vi "Motion@WaitPathIndex__Parameter.vi"(1 "ParamterIn":string) -> (0 "ParamterOut":string)   [LabVIEW 2020]
panel:
  in  "Message=":string(combo)
  in  "TimeOut=":string(combo)
  in  "Parameter":string(combo)
  in  "MotorName":string(combo)
  in  "Confirm":bool
  # "Motion@WaitPathIndex $Motor,$Index(,TimeOut=XXX,Message=XXX)"
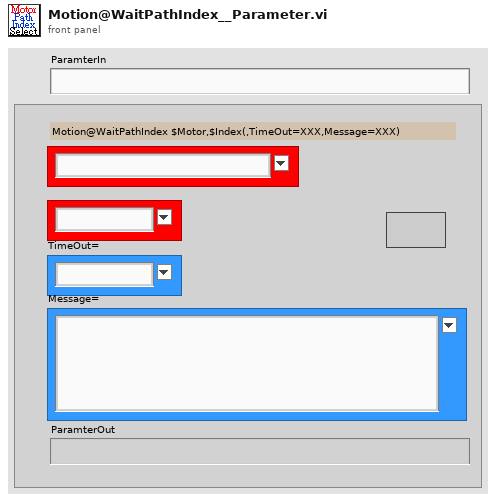
[diagram p1: front panel]
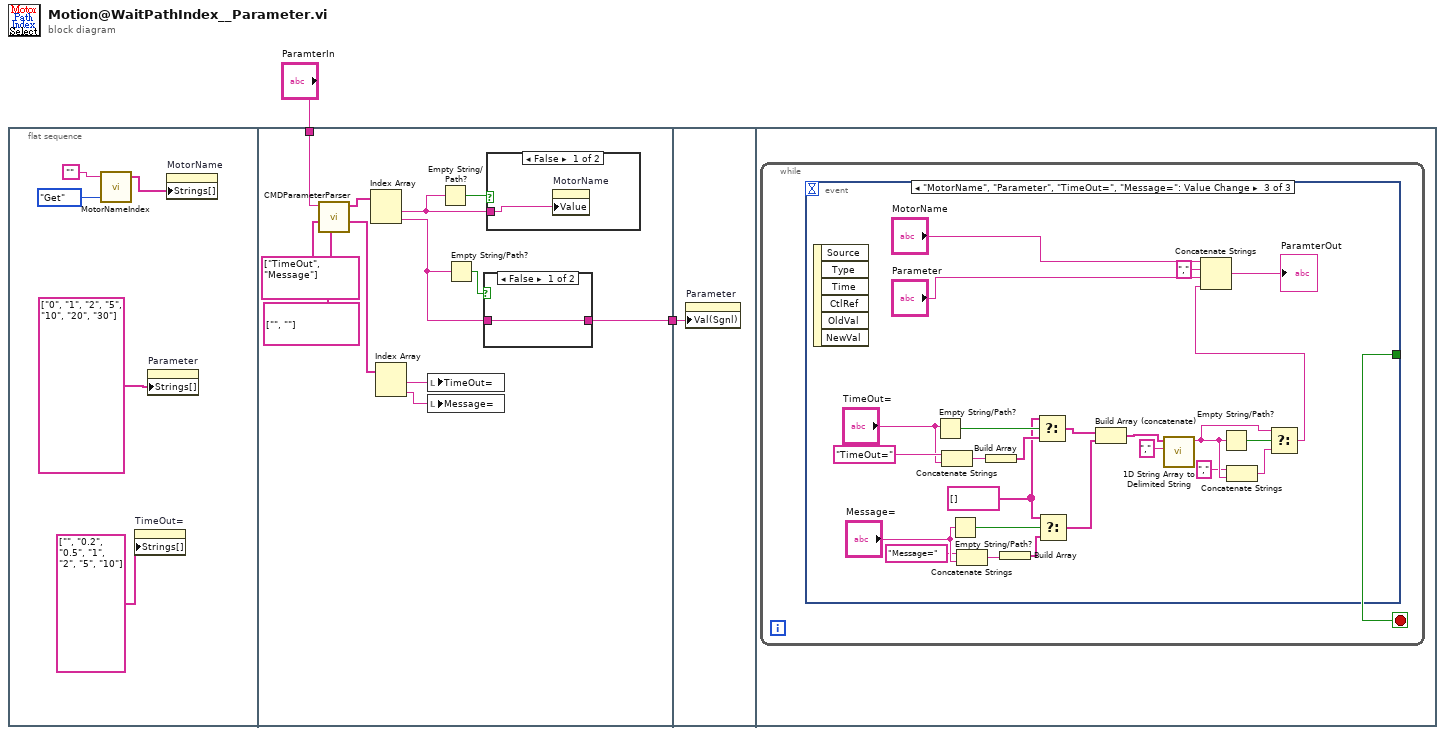
[diagram p0: block diagram]
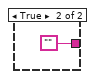
[diagram p2: hidden frame]
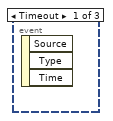
[diagram p4: hidden frame]
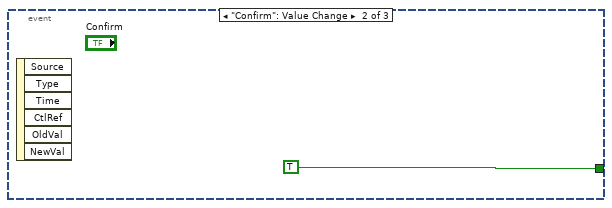
[diagram p5: hidden frame]
diagram:
  n1 = flat-sequence {
    tunnel: "ParamterIn" -> [w16]
    tunnel: [w17] -> w1
    tunnel: w1 -> [w23]
    frame #0 {
      n2 = call "MotorNameIndex.vi"("OP"=enum16{"Get", "Update", "Init"}."Get", "MotorName"="") -> ("MotorList"=w5:string[])  [unwired: 1 in, 2 out]
      n3 = property on="TimeOut=" class="CmbBox"("Strings[]"=string[] ["", "0.2", "0.5", "1", "2", "5", "10"] ("Strings []")) -> ()  [unwired: 2 in, 2 out]
      n4 = property on="Parameter" class="CmbBox"("Strings[]"=string[] ["0", "1", "2", "5", "10", "20", "30"] ("Strings []")) -> ()  [unwired: 2 in, 2 out]
      n5 = property on="MotorName" class="CmbBox"("Strings[]"=w5) -> ()  [unwired: 2 in, 2 out]
    }
    frame #1 {
      n6 = call "CMDParameterParser.vi"("DeafultValues"=string[] ["", ""], "RequiredKeys"=string[] ["TimeOut", "Message"], "CMDParameter"=w16) -> ("KeyValues"=w10:string[], "Input"=w15:string[])  [unwired: 6 in, 1 out]
      n7 = Index Array(array=w15) -> (element #1=w14:string, element #2=w13:string)  [unwired: 2 in]
      n8 = Index Array(array=w10) -> (element #1=w9:string, element #2=w8:string)  [unwired: 2 in]
      n9 = local write "TimeOut="(w9) -> ()
      n10 = local write "Message="(w8) -> ()
      n11 = Empty String/Path?(string/path=w14) -> (empty?=w19:bool)
      n12 = Empty String/Path?(string/path=w13) -> (empty?=w18:bool)
      n13 = case shown="False" w18 {
        tunnel: [w20 ""] -> w17
        tunnel: w13 -> [w20 _]
        frame False {
        }
        frame True {
        }
      }
      n14 = case shown="False" w19 {
        tunnel: w14 -> [w22 _]
        frame False {
          n15 = property on="MotorName" class="CmbBox"("Value"=w22) -> ()  [unwired: 2 in, 2 out]
        }
        frame True {
        }
      }
    }
    frame #2 {
      n16 = property on="Parameter" class="CmbBox"("Val(Sgnl)"=w23) -> ()  [unwired: 2 in, 2 out]
    }
    frame #3 {
      n17 = while {
        stop <- w24 stop-if-true
        n18 = event shown="[2] \"MotorName\", \"Parameter\", \"TimeOut=\", \"Message=\": Value Change" {
          selector: _ -> [_ _ _]
          dyn-events: _ -> [_ _ _]
          timeout: _ -> [_ _ _]
          tunnel: [_ TRUE _] -> w24
          event Timeout {
            n19 = event-data() -> ()  [unwired: 1 in, 3 out]
          }
          event "Confirm": Value Change {
            n20 = event-data() -> ()  [unwired: 1 in, 6 out]
          }
          event "MotorName", "Parameter", "TimeOut=", "Message=": Value Change {
            w41 = string[] [] ("t")
            n21 = event-data() -> ()  [unwired: 1 in, 6 out]
            n22 = Empty String/Path?(string/path="TimeOut=") -> (empty?=w47:bool)
            n23 = Concatenate Strings("TimeOut=" ("string"), "TimeOut=") -> (w45:string)
            n24 = Empty String/Path?(string/path="Message=") -> (empty?=w46:bool)
            n25 = Concatenate Strings("Message=" ("string"), "Message=") -> (w43:string)
            n26 = Build Array(w45) -> (w44:string[])
            n27 = Build Array(w43) -> (w42:string[])
            n28 = Select(t=w41, s=w47, f=w44) -> (s? t:f=w40:string[])
            n29 = Select(t=w41, s=w46, f=w42) -> (s? t:f=w39:string[])
            n30 = Build Array (concatenate)(w40, w39) -> (w33:string[])
            n31 = call <vilib>:"1D String Array to Delimited String.vi"("delimiter"=",", "string array"=w33) -> ("delimited string"=w36:string)  [unwired: 9 in]
            n32 = Empty String/Path?(string/path=w36) -> (empty?=w37:bool)
            n33 = Concatenate Strings("," ("string"), w36) -> (w34:string)
            n34 = Select(t=w36, s=w37, f=w34) -> (s? t:f=w26:string)
            n35 = Concatenate Strings("MotorName", "," ("string"), "Parameter", w26) -> (→"ParamterOut":string)
          }
        }
      }
    }
  }
